vi "MTM2_logEvent_m2FaultState.vi"(8 "error in (no error)":errorcluster, 11 "logevent_m2FaultState_Ctl":T1) -> (0 "error out":errorcluster, 2 "function return":i32, 3 "logevent_m2FaultState_Ctl out":T1)   [LabVIEW 2018, in "SALLV_MTM2.lvlib"]
doc: "int MTM2_shm_logEvent_m2FaultStateLV(MTM2_logevent_m2FaultStateLV *logevent_m2FaultState_Ctl );"
uses:
  SALLV_MTM2.lvlib
  DataTypes/logevent_m2FaultState.ctl
  SALLV_MTM2.so
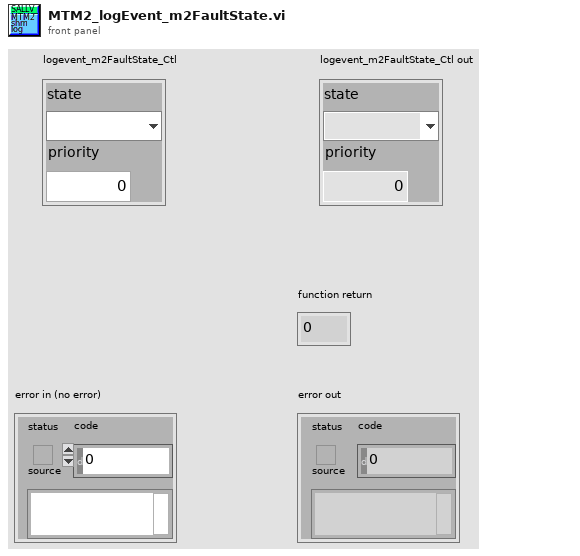
[diagram p1: front panel]
types:
  T1 = typedef "SALLV_MTM2.lvlib/logevent_m2FaultState.ctl" = cluster{"state":enum32{"", "ActuatorPlusLimit", "ActuatorMinusLimit", "ActuatorPlusForceLimit", "ActuatorMinusForceLimit", "ActuatorCommTimeout", "FollowingError", "ConfigurationError", "UnresponsiveActuator", "TangentLinkStrainFault", "cRIOCommFailure", "cRIOHeartbeatFailure", "CurrentError", "VoltageError", "PowerRelayFault", "PowerSupplyFault", "TemperatureFault", "TempSensorFailure", "TelescopeElevationFault", "GravitySensorFailure", "ILCFault", "CelRBPositionError", "DisplacementSensor", "ActuatorPlusSoftLimit", "ActuatorMinusSoftLimit", "CelTemperatureWarning"}, "priority":i32}
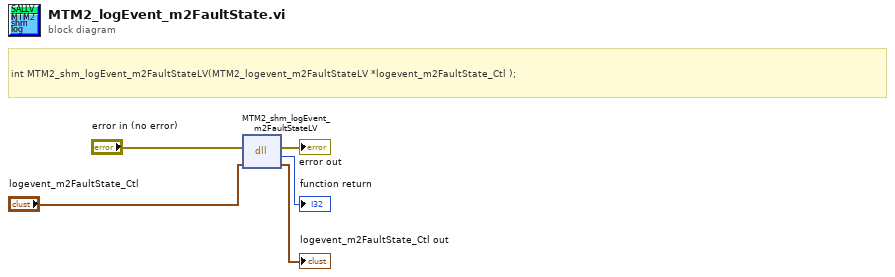
[diagram p0: block diagram]
diagram:
  # "int MTM2_shm_logEvent_m2FaultStateLV(MTM2_logevent_m2FaultStateLV *logevent_m2FaultState_Ctl );"
  n1 = dll-call lib="home/ttsai/Document/salApiMTM2/SALLV_MTM2/SALLV_MTM2.*" fn="MTM2_shm_logEvent_m2FaultStateLV"(error in="error in (no error)", "logevent_m2FaultState_Ctl"="logevent_m2FaultState_Ctl") -> (error out=→"error out":errorcluster, →"function return":i32, "logevent_m2FaultState_Ctl"=→"logevent_m2FaultState_Ctl out":T1)  [unwired: 2 in, 1 out]
